vi "__anritsu_simple_read.vi"() -> ()   [LabVIEW 2013]
panel:
  out "sum":dbl
  in  "Take Away Background?":bool=TRUE
  in  "Power dBm":dbl[](graph)
  in  "Frequency choice":bool
  in  "Tab Control 2":enum32{"A", "B"}(tab)
  in  "F_end (Hz)":dbl=10000000.0 min=0.0 format="%#_13p"
  in  "F_begin (Hz)":dbl format="%#_13p"
  in  "Center (Hz)":dbl min=0.0 format="%#_13p"
  in  "Span (Hz)":dbl=10000000.0 min=0.0 format="%#_13p"
  in  "Tab Control":enum32{"Page 1"}(tab)
  in  "Boolean":bool=TRUE
  in  "Name":string="data_labview_spa_9Mar'19_niAmplifier"
  out "Power dBm":dbl[](graph)
  out "Measurment time (s)":dbl=197.0
  in  "Points":i32=1001 min=1 max=10001 step=1
  in  "VBW (Hz)":dbl=30.0 format="%#_13g"
  in  "RBW (Hz)":dbl=1000.0 format="%#_13p"
  # "BACKGROUND"
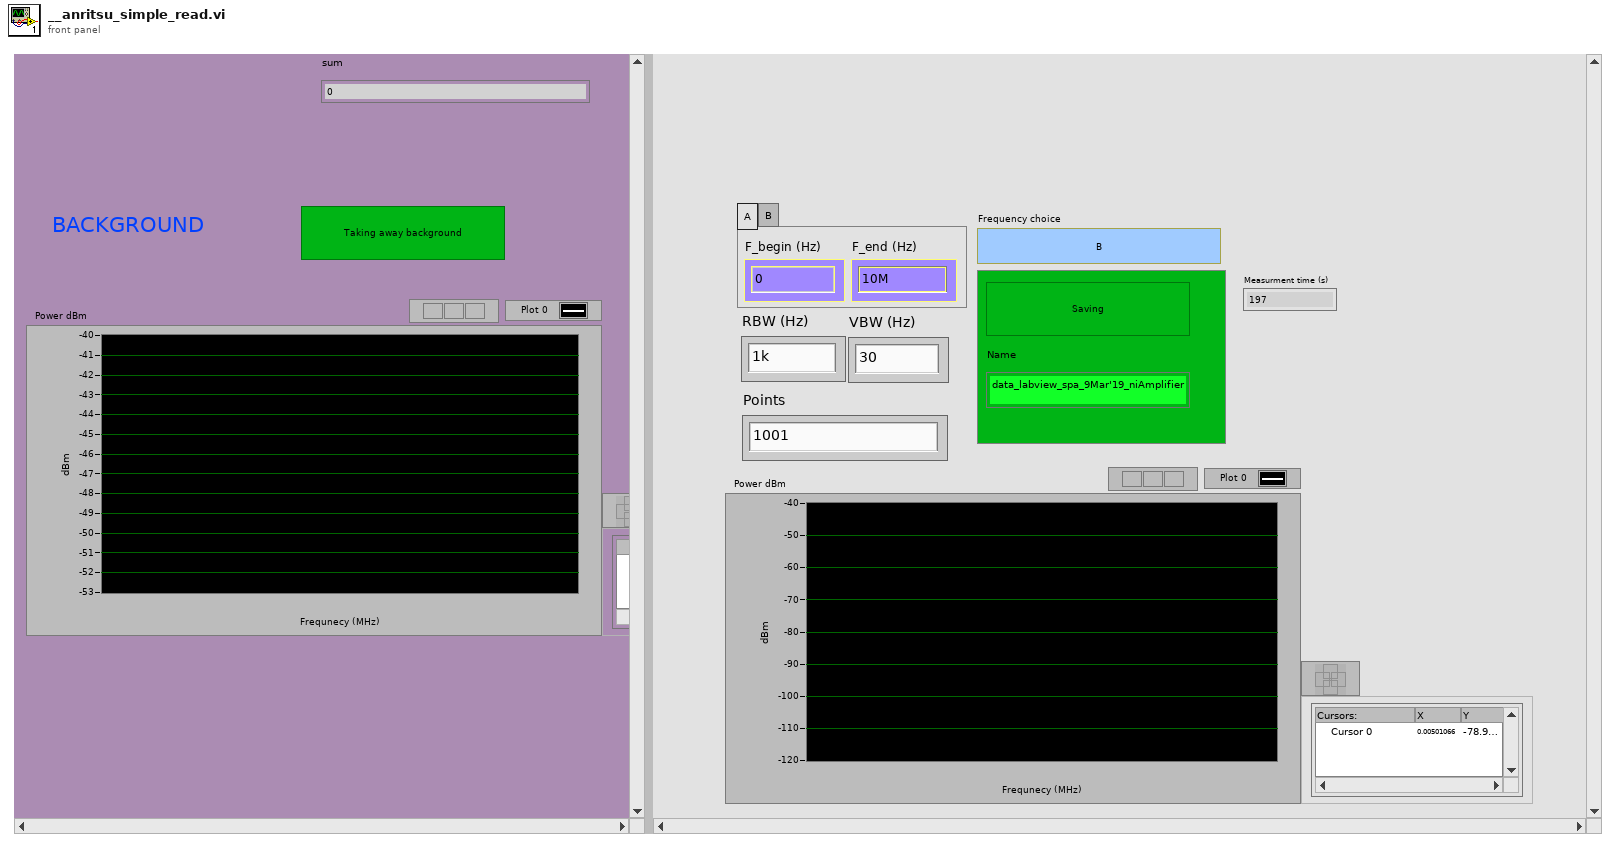
[diagram p1: front panel]
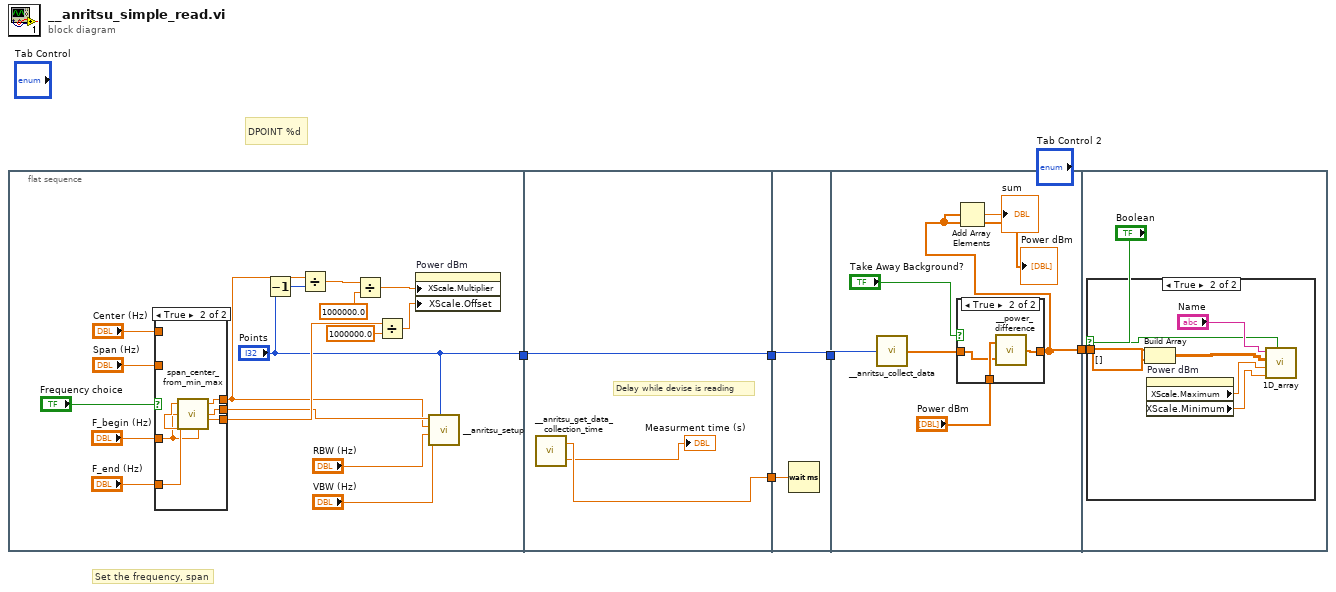
[diagram p0: block diagram]
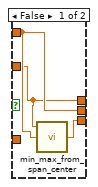
[diagram p2: hidden frame]
diagram:
  # "Set the frequency, span"
  # "DPOINT %d"
  n1 = flat-sequence {
    tunnel: ["Points"] -> w5
    tunnel: w5 -> [w32]
    tunnel: [w31] -> w4
    tunnel: [w32] -> w2
    tunnel: w4 -> [w34]
    tunnel: [w33] -> w3
    tunnel: w2 -> [w33]
    tunnel: w3 -> [w38]
    tunnel: [w36] -> w1
    tunnel: w1 -> [w45]
    frame #0 {
      n2 = case shown="True" "Frequency choice" {
        tunnel: [w25 w26] -> w10
        tunnel: "F_begin (Hz)" -> [_ w28]
        tunnel: "F_end (Hz)" -> [_ w29]
        tunnel: [w24 w27] -> w9
        tunnel: "Span (Hz)" -> [w24 _]
        tunnel: "Center (Hz)" -> [w25 _]
        tunnel: [w23 w28] -> w11
        frame False {
          n3 = call "min_max_from_span_center.vi"("Mid Point"=w25, "Span"=w24) -> ("Start"=w23:dbl)  [unwired: 1 in, 2 out]
        }
        frame True {
          n4 = call "span_center_from_min_max.vi"("Begin"=w28, "End"=w29) -> ("Mid Point"=w26:dbl, "Difference (abs)"=w27:dbl)  [unwired: 1 in, 1 out]
        }
      }
      n5 = Decrement(x="Points") -> (x-1=w19:i32)
      n6 = Divide(x=w9, y=w19) -> (x/y=w20:dbl)
      n7 = Divide(x=w20, y=1000000.0) -> (x/y=w22:dbl)
      n8 = Divide(x=w11, y=1000000.0) -> (x/y=w12:dbl)
      n9 = property on="Power dBm" class="WFGraph (strict)"("XScale.Multiplier"=w22, "XScale.Offset"=w12) -> ()  [unwired: 2 in, 2 out]
      n10 = call "__anritsu_setup.vi"("Center Freq (Hz)"=w10, "Span (Hz)"=w9, "RBW (Hz)"="RBW (Hz)", "VBW (Hz)"="VBW (Hz)", "Points"="Points") -> ()  [unwired: 1 out]
    }
    frame #1 {
      # "Delay while devise is reading"
      n11 = call "__anritsu_get_data_collection_time.vi"() -> ("Measurment time (s)"=→"Measurment time (s)":dbl, "Time to wait (ms)"=w31:dbl)
    }
    frame #2 {
      n12 = Wait (ms)(milliseconds to wait=w34) -> ()  [unwired: 1 out]
    }
    frame #3 {
      n13 = call "__anritsu_collect_data.vi"("Points to read"=w38) -> ("Data out"=w37:dbl[])
      n14 = case shown="True" "Take Away Background?" {
        tunnel: [w41 w44] -> w36
        tunnel: w37 -> [w41 w42]
        tunnel: "Power dBm" -> [_ w43]
        frame False {
        }
        frame True {
          n15 = call "__power_difference.vi"("Power Low dBm"=w42, "Power High dBm"=w43) -> ("Power Difference dBm"=w44:dbl[])
        }
      }
      "Power dBm" <- w36
      n16 = Add Array Elements(numeric array=w36) -> (sum=→"sum":dbl)
    }
    frame #4 {
      n17 = case shown="True" "Boolean" {
        selector: "Boolean" -> [_ w50]
        tunnel: w45 -> [_ w53]
        frame False {
        }
        frame True {
          n18 = Build Array(w53, dbl[] [] ("element")) -> (w49:dbl[][])
          n19 = property on="Power dBm" class="WFGraph (strict)"() -> ("XScale.Maximum"=w48:dbl, "XScale.Minimum"=w47:dbl)  [unwired: 2 in, 2 out]
          n20 = call "1D_array.vi"("Name"="Name", "Array"=w49, "x_max"=w48, "x_min"=w47, "Save?"=w50) -> ()  [unwired: 1 out]
        }
      }
    }
  }
